vi "ConvertADCReading.vi"(2 "Reading / V":dbl format="%#_13g", 3 "Input arm settings":T1={"Vref"=1.0, "Rgain"=100000.0, "Rset"=10000.0, "Rseries"=1000.0, "Input polarity?"=FALSE}) -> (0 "Voltage / V":dbl=nan, 1 "Temperature / C":dbl=nan format="%0.2f")   [LabVIEW 2015]
doc: "Converts a reading from the controller in volts into a temperature using the given parameters"
uses:
  <vilib>/imath/engines/lvmath2/RunTimeEngine/ArithmeticOperatorToken/NIMS_ArithmeticOperator_power(S).vi
  <instcachedir>/0/NIMS_ArithmeticOperator_power(S)_DFB67823F1414E5097C86E39787D8CA8.lvgen/NIMS_ArithmeticOperator_power(S)_DFB67823F1414E5097C86E39787D8CA8_010.vi
  <vilib>/imathl/engines/lvmath/Functions/Error Handling/Create Error.vi
  <vilib>/imath/engines/lvmath2/RunTimeEngine/NodeEndStatement/NIMS_NodeEndStatement_Output.vi
  <instcachedir>/0/NIMS_NodeEndStatement_Output_53EC0D466D134D7ABD903AC30B43404B.lvgen/NIMS_NodeEndStatement_Output_53EC0D466D134D7ABD903AC30B43404B_001.vi
  <instcachedir>/0/NIMS_NodeEndStatement_Output_53EC0D466D134D7ABD903AC30B43404B.lvgen/NIMS_NodeEndStatement_Output_53EC0D466D134D7ABD903AC30B43404B_009.vi
  <vilib>/imath/engines/lvmath2/RunTimeEngine/ErrorHandling/NIMS_Finalize Error.vi
panel:
  out "Rtherm":dbl=nan
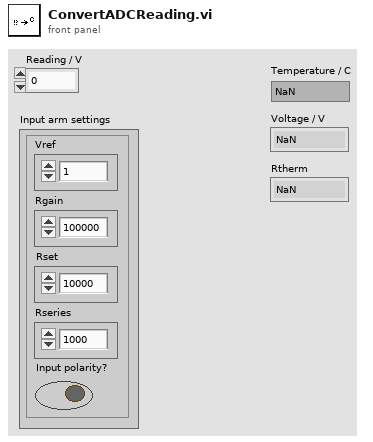
[diagram p1: front panel]
types:
  T1 = cluster{"Vref":dbl, "Rgain":dbl, "Rset":dbl, "Rseries":dbl, "Input polarity?":bool}
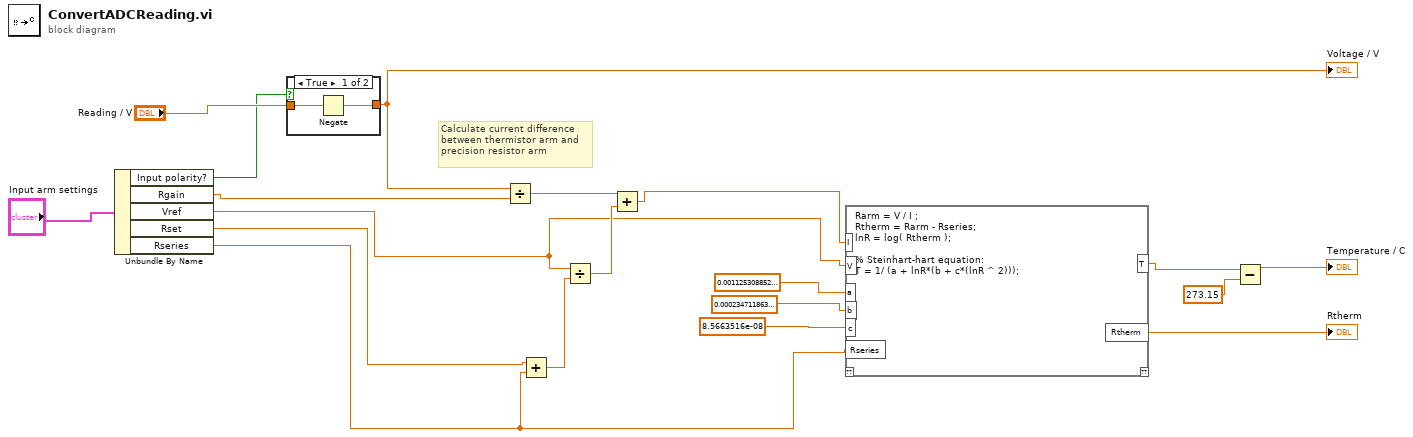
[diagram p0: block diagram]
diagram:
  # "Calculate current difference\nbetween thermistor arm and\nprecision resistor arm"
  n1 = Unbundle By Name("Input arm settings") -> ("Input polarity?"=w6:bool, "Rgain"=w5:dbl, "Vref"=w4:dbl, "Rset"=w2:dbl, "Rseries"=w3:dbl)
  n2 = case shown="True" w6 {
    tunnel: [w20 w22] -> w7
    tunnel: "Reading / V" -> [w21 w22]
    frame True {
      n3 = Negate(x=w21) -> (-x=w20:dbl)
    }
    frame False {
    }
  }
  "Voltage / V" <- w7
  n4 = Divide(x=w7, y=w5) -> (x/y=w19:dbl)
  n5 = Add(x=w2, y=w3) -> (x+y=w14:dbl)
  n6 = Divide(x=w4, y=w14) -> (x/y=w18:dbl)
  n7 = Add(x=w19, y=w18) -> (x+y=w12:dbl)
  n8 = mathscript code="Rarm = V / I ;\nRtherm = Rarm - Rseries;\nlnR = log( Rtherm );\n\n% Steinhart-hart equation:\nT = 1/ (a + lnR*(b + c*(lnR ^ 2)));"("I"=w12, "V"=w4, "a"=0.001125308852122, "b"=0.000234711863267, "c"=8.5663516e-08, "Rseries"=w3) -> ("T"=w13:cdb, "Rtherm"=→"Rtherm":dbl)  [unwired: 1 in, 1 out]
  n9 = Subtract(x=w13, y=273.15) -> (x-y=→"Temperature / C":cdb)
